vi "Close.vi"(8 "error in (no error)":errorcluster, 11 "Controller in":T1) -> (0 "error out":errorcluster)   [LabVIEW 2017, in "Roboteq Controller KBL1xxx.lvlib"]
doc: "Performs termination the software connection to the instrument."
uses:
  <instrlib>/Roboteq Controller KBL1xxx/Roboteq Controller KBL1xxx.lvlib
  <instrlib>/Roboteq Controller KBL1xxx/Public/Controls/Controller.ctl
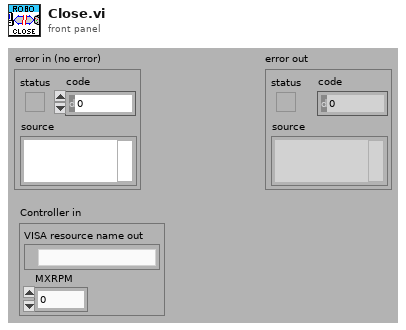
[diagram p1: front panel]
types:
  T1 = typedef "Roboteq Controller KBL1xxx.lvlib/Controller.ctl" = cluster{"VISA resource name out":refnum<visa-resource-name>, "MXRPM":u16}
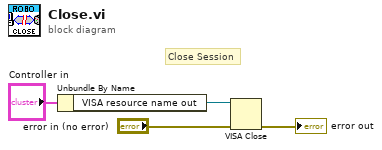
[diagram p0: block diagram]
diagram:
  # "Close Session"
  n1 = Unbundle By Name("Controller in") -> ("VISA resource name out"=w1:refnum<visa-resource-name>)
  n2 = VISA Close(VISA resource name=w1, error in (no error)="error in (no error)") -> (error out=→"error out":errorcluster)
